vi "default colors.vi"(11 "colors":T1) -> (3 "default color":T1)   [LabVIEW 2021, in "RocketPlot.lvlib" / "TipTablePanel.lvclass"]
uses:
  TipTablePanel.lvclass
  colors.ctl
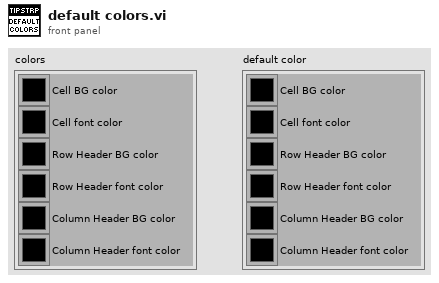
[diagram p1: front panel]
types:
  T1 = typedef "RocketPlot.lvlib/TipTablePanel.lvclass/colors.ctl" = cluster{"Cell BG color":u32, "Cell font color":u32, "Row Header BG color":u32, "Row Header font color":u32, "Column Header BG color":u32, "Column Header font color":u32}
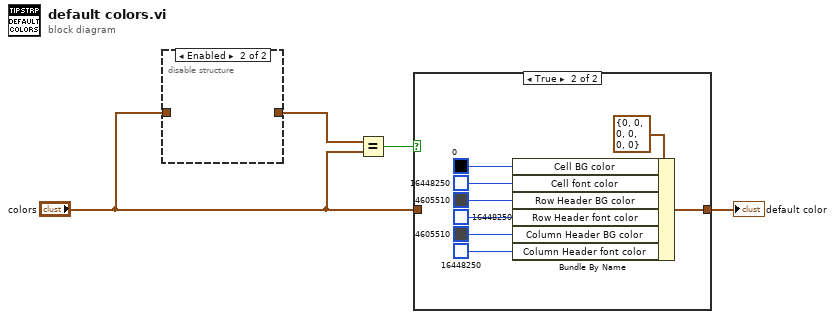
[diagram p0: block diagram]
diagram:
  n1 = disable-structure shown="Enabled" {
    disable-tunnel: "colors" -> [w5 _]
    disable-tunnel: [w5 _] -> w3
    frame Disabled {
    }
    frame Enabled {
    }
  }
  n2 = Equal?(x=w3, y="colors") -> (x = y?=w2:bool)
  n3 = case shown="True" w2 {
    tunnel: [w6 w13] -> w4
    tunnel: "colors" -> [w6 _]
    frame False {
    }
    frame True {
      n4 = Bundle By Name(cluster=T1 {"Cell BG color"=0, "Cell font color"=0, "Row Header BG color"=0, "Row Header font color"=0, "Column Header BG color"=0, "Column Header font color"=0} ("default color"), "Cell BG color"=u32 0, "Cell font color"=u32 16448250, "Row Header BG color"=u32 4605510, "Row Header font color"=u32 16448250, "Column Header BG color"=u32 4605510, "Column Header font color"=u32 16448250) -> (w13:T1)
    }
  }
  "default color" <- w4
